vi "DemoClient.vi"(8 "Error In":errorcluster, 10 "Data":variant, 11 "Queues":T1) -> ()   [LabVIEW 2017, in "Client.lvlib"]
uses:
  Client.lvlib
  ServerLib/SubLibs/Message Queue/CommReferences.ctl
  ServerLib/SubLibs/Message Queue/MessageCluster.ctl
  TypeDefs/SR List.ctl
  TypeDefs/SR Data.ctl
  <vilib>/httpClient/LabVIEWHTTPClient.lvlib
  ServerLib/SubLibs/Message Queue/Message Queue.lvlib
panel:
  out "SRs":string[][](table)
  out "HeartbeatBody":string
  out "HeartbeatHeader":string
  out "SRheader":string
  out "SRbody":string
  out "GetSR-Error":errorcluster
  in  "UpdateSRs":bool
  in  "Heartbeat Period (s)":dbl=10.0 format="%#_13g"
  in  "ClientName":string="TestClient"
  in  "Port":string="8001"
  in  "IP":string="localhost"
  out "HeartbeatError":errorcluster
  in  "Stop Button":bool
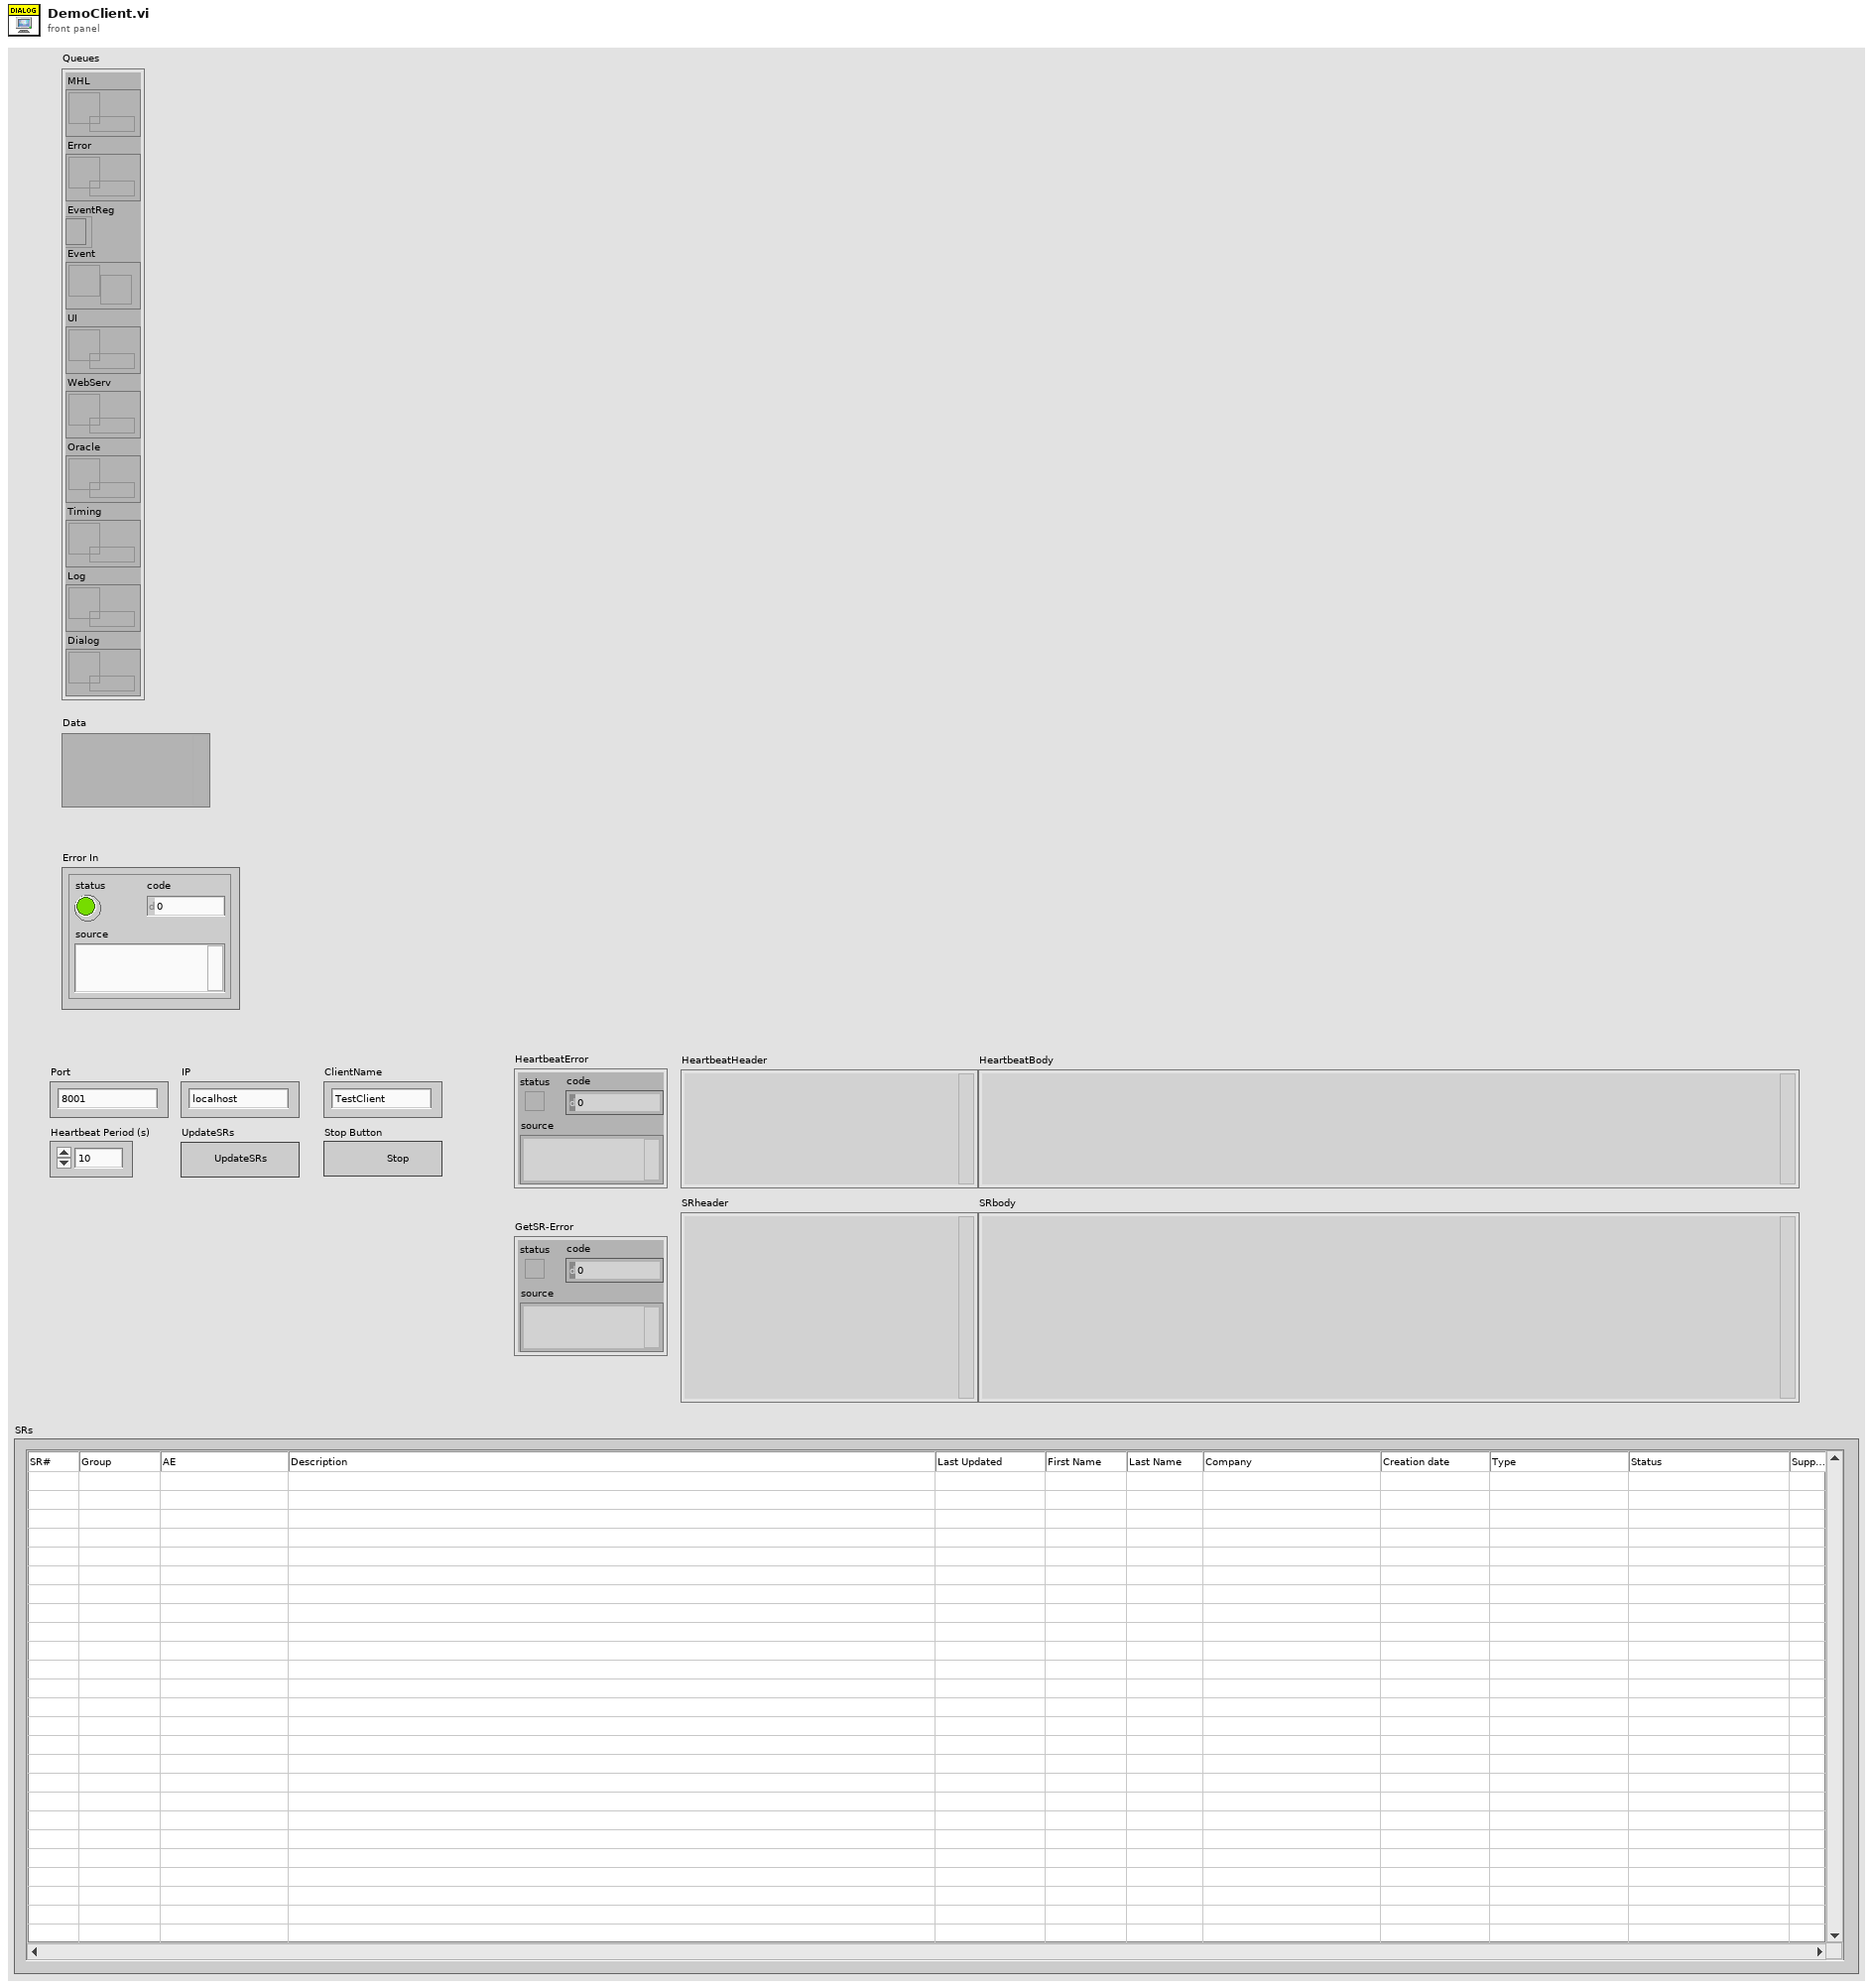
[diagram p1: front panel]
types:
  T1 = typedef "Server.lvlib/Message Queue.lvlib/CommReferences.ctl" = cluster{"MHL":refnum<queue>, "Error":refnum<queue>, "EventReg":refnum<event-registration>, "Event":refnum<user-event>, "UI":refnum<queue>, "WebServ":refnum<queue>, "Oracle":refnum<queue>, "Timing":refnum<queue>, "Log":refnum<queue>, "Dialog":refnum<queue>}
  T2 = cluster{"IP":string, "Port":string, "ClientName":string}
  T3 = typedef "Client.lvlib/SR List.ctl" = T4[]
  T4 = typedef "Client.lvlib/SR Data.ctl" = cluster{"SR#":dbl, "Group":string, "Owner":string, "Problem Summary":string, "Last Updated":timestamp, "Customer First Name":string, "Customer Last Name":string, "Company":string, "Created On":timestamp, "SR Type":string, "Status":string, "Service Level":string, "Channel":string, "Days Open":dbl}
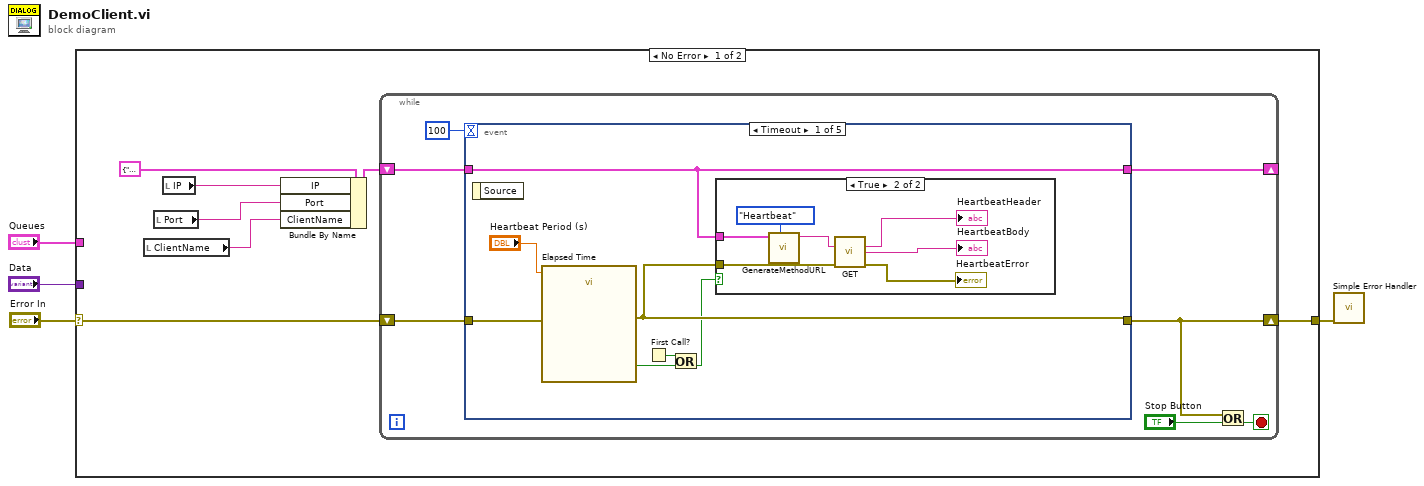
[diagram p0: block diagram]
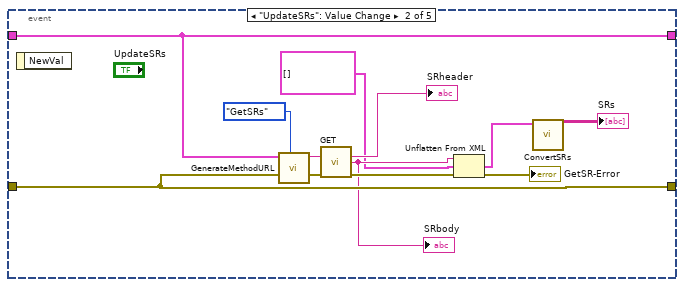
[diagram p3: hidden frame]
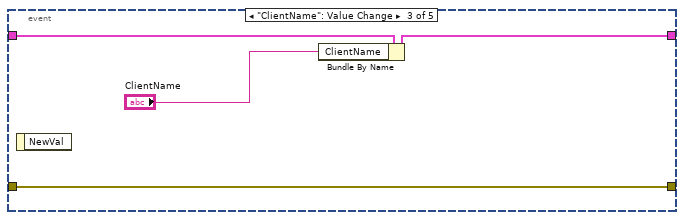
[diagram p4: hidden frame]
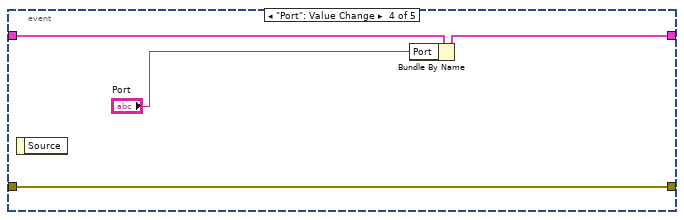
[diagram p5: hidden frame]
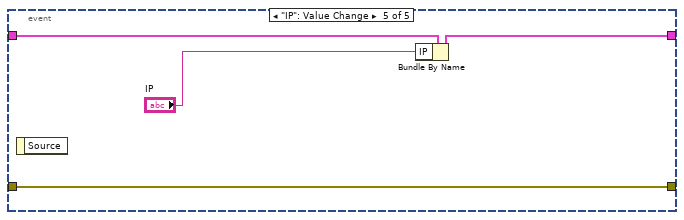
[diagram p6: hidden frame]
diagram:
  n1 = case shown="No Error" "Error In" {
    selector: "Error In" -> [w11 w56]
    tunnel: [w10 w56] -> w1
    tunnel: "Queues" -> [_ _]
    tunnel: "Data" -> [_ _]
    frame No Error {
      n2 = local read "ClientName"() -> (w5:string)
      n3 = local read "Port"() -> (w7:string)
      n4 = local read "IP"() -> (w6:string)
      n5 = Bundle By Name(cluster=T2 {"IP"="", "Port"="", "ClientName"=""}, "IP"=w6, "Port"=w7, "ClientName"=w5) -> (w8:T2)
      n6 = while {
        shift-right: [w15] -> w10
        shift-left: w11 -> [w18]
        shift-right: [w13] -> _
        shift-left: w8 -> [w12]
        stop <- w16 stop-if-true
        n7 = event shown="[0] Timeout" {
          selector: _ -> [_ _ _ _ _]
          dyn-events: _ -> [_ _ _ _ _]
          timeout: 100 -> [_ _ _ _ _]
          tunnel: w18 -> [w25 w37 w47 w50 w55]
          tunnel: [w24 w37 w47 w50 w55] -> w15
          tunnel: [w22 w43 w45 w49 w53] -> w13
          tunnel: w12 -> [w22 w43 w46 w51 w54]
          event Timeout {
            n8 = event-data() -> ()  [unwired: 1 in, 1 out]
            n9 = call "Elapsed Time"("Time Target (s)"="Heartbeat Period (s)", "error in (no error)"=w25) -> ("Time has Elapsed"=w23:bool, "error out"=w24:errorcluster)  [unwired: 10 in, 6 out]
            n10 = First Call?() -> (First Call?: T/F=w19:bool)
            n11 = Or(x=w19, y=w23) -> (x .or. y?=w20:bool)
            n12 = case shown="True" w20 {
              tunnel: w24 -> [_ w31]
              tunnel: w22 -> [_ w30]
              frame False {
              }
              frame True {
                n13 = call "GenerateMethodURL.vi"("Method"=enum16{"Heartbeat", "GetSRs"}."Heartbeat", "TestClientData"=w30) -> ("String"=w29:string)  [unwired: 9 in]
                n14 = call <vilib>:"GET.vi"("url"=w29, "error in (no error)"=w31) -> ("headers"=→"HeartbeatHeader":string, "body"=→"HeartbeatBody":string, "error out"=→"HeartbeatError":errorcluster)  [unwired: 10 in, 1 out]
              }
            }
          }
          event "UpdateSRs": Value Change {
            n15 = event-data() -> ()  [unwired: 1 in, 1 out]
            n16 = call "GenerateMethodURL.vi"("Method"=enum16{"Heartbeat", "GetSRs"}."GetSRs", "TestClientData"=w43) -> ("String"=w41:string)  [unwired: 9 in]
            n17 = call <vilib>:"GET.vi"("url"=w41, "error in (no error)"=w37) -> ("headers"=→"SRheader":string, "body"=w36:string, "error out"=w38:errorcluster)  [unwired: 10 in, 1 out]
            "SRbody" <- w36
            n18 = Unflatten From XML(xml string=w36, type=T3 [] ("SRList"), error in (no error)=w38) -> (value=w34:T3, error out=→"GetSR-Error":errorcluster)
            n19 = call "ConvertSRs.vi"("SRList"=w34) -> ("SRlistString"=→"SRs":string[][])  [unwired: 10 in]
          }
          event "ClientName": Value Change {
            n20 = event-data() -> ()  [unwired: 1 in, 1 out]
            n21 = Bundle By Name(cluster=w46, "ClientName"="ClientName") -> (w45:T2)
          }
          event "Port": Value Change {
            n22 = event-data() -> ()  [unwired: 1 in, 1 out]
            n23 = Bundle By Name(cluster=w51, "Port"="Port") -> (w49:T2)
          }
          event "IP": Value Change {
            n24 = event-data() -> ()  [unwired: 1 in, 1 out]
            n25 = Bundle By Name(cluster=w54, "IP"="IP") -> (w53:T2)
          }
        }
        n26 = Or(x=w15, y="Stop Button") -> (x .or. y?=w16:bool)
      }
    }
    frame Error {
    }
  }
  n27 = call <vilib>:"Simple Error Handler.vi"("error in (no error)"=w1) -> ()  [unwired: 4 in, 5 out]
